vi "donut Animate.vi"() -> ()   [LabVIEW 2012]
doc: "This VI demonstrates how to animate a picture on the front panel using a picture ring (Pict Ring) control. This VI takes a sequence of pictures where each picture represents a \"frame\" of the animaction and makes each picture a selection in the picture ring. By programmatically incrementing the value of the picture ring, the picture appears to be animated."
panel:
  in  "Frames Per Second":u32(slide)=30 scale=1.0..60.0
  in  "stop":bool
  out "Picture Ring":u16(ring)
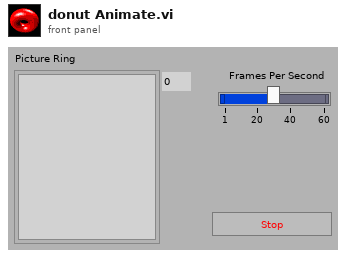
[diagram p1: front panel]
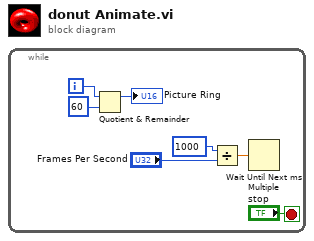
[diagram p0: block diagram]
diagram:
  n1 = while {
    i -> [w7]
    stop <- "stop" stop-if-true
    n2 = Quotient & Remainder(x=w7, y=60) -> (x-y*floor(x/y)=→"Picture Ring":i32)  [unwired: 1 out]
    n3 = Divide(x=u32 1000, y="Frames Per Second") -> (x/y=w1:dbl)
    n4 = Wait Until Next ms Multiple(millisecond multiple=w1) -> ()  [unwired: 1 out]
  }
